vi "UpdateROI.vi"(6 "value":u16, 8 "error in (no error)":errorcluster, 9 "ElementToUpdate":string, 11 "Photometrics Cam v2 in":refnum<class "Photometrics_CH-250_Cam.lvclass">) -> (0 "error out":errorcluster, 3 "Photometrics Cam v2 out":refnum<class "Photometrics_CH-250_Cam.lvclass">)   [LabVIEW 2013, in "Photometrics_CH-250_Cam.lvclass"]
uses:
  Photometrics_CH-250_Cam.lvclass
  CameraSessionClass/CS250-CameraHardwareClass.lvclass
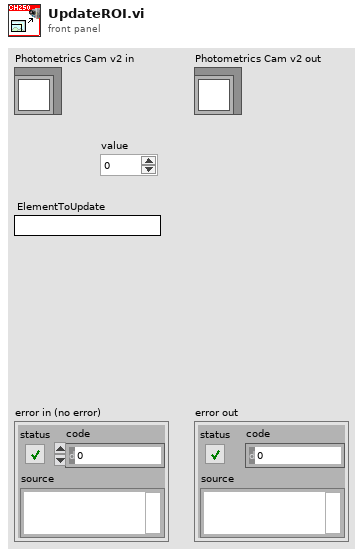
[diagram p1: front panel]
types:
  T1 = typedef "ROI_TypDef.ctl" = cluster{"Width":cluster{"Value":dbl, "Min":dbl, "Max":dbl, "StepSize":dbl, "Tolerance":dbl, "valueactual":dbl}, "Height":cluster{"Value":dbl, "Min":dbl, "Max":dbl, "StepSize":dbl, "Tolerance":dbl, "valueactual":dbl}, "OffsetX":cluster{"Value":dbl, "Min":dbl, "Max":dbl, "StepSize":dbl, "Tolerance":dbl, "valueactual":dbl}, "OffsetY":cluster{"Value":dbl, "Min":dbl, "Max":dbl, "StepSize":dbl, "Tolerance":dbl, "valueactual":dbl}}
  T2 = cluster{"s1":u16, "s2":u16, "sbin":u16, "p1":u16, "p2":u16, "pbin":u16}
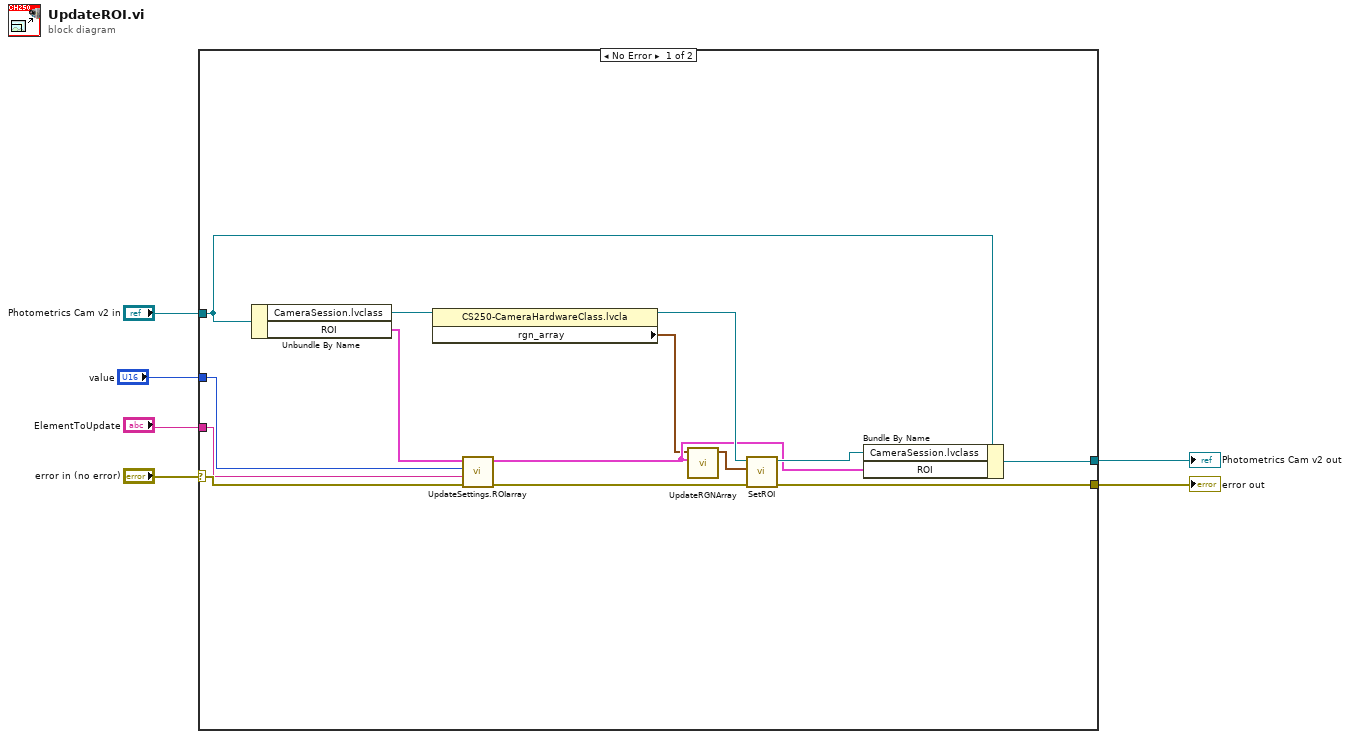
[diagram p0: block diagram]
diagram:
  n1 = case shown="No Error" "error in (no error)" {
    selector: "error in (no error)" -> [w17 w22]
    tunnel: [w20 w21] -> w6
    tunnel: "Photometrics Cam v2 in" -> [w19 w21]
    tunnel: [w18 w22] -> w4
    tunnel: "ElementToUpdate" -> [w11 _]
    tunnel: "value" -> [w10 _]
    frame No Error {
      n2 = Unbundle By Name(w19) -> ("CameraSession.lvclass"=w13:refnum<class "CS250-CameraHardwareClass.lvclass">, "ROI"=w14:T1)
      n3 = property class="CS250-CameraHardwareClass.lvcla"(reference=w13) -> (reference out=w12:refnum<class "CS250-CameraHardwareClass.lvclass">, "rgn_array"=w7:T2)  [unwired: 1 in, 1 out]
      n4 = call "UpdateSettings.ROIarray.vi"("error in (no error)"=w17, "ElementToUpdate"=w11, "value"=w10, "ROI in"=w14) -> ("error out"=w16:errorcluster, "ROI out"=w8:T1)  [unwired: 6 in]
      n5 = call "UpdateRGNArray.vi"("NewROI"=w8, "rgn_array in"=w7) -> ("rgn_array out"=w15:T2)  [unwired: 9 in]
      n6 = call-dynamic "SetROI.vi"("error in (no error)"=w16, "NewROI"=w15, "CameraSession in"=w12) -> ("error out"=w18:errorcluster, "CameraSession out"=w9:refnum<class "CS250-CameraHardwareClass.lvclass">)  [unwired: 7 in]
      n7 = Bundle By Name(cluster=w19, "CameraSession.lvclass"=w9, "ROI"=w8) -> (w20:refnum<class "Photometrics_CH-250_Cam.lvclass">)
    }
    frame Error {
    }
  }
  "Photometrics Cam v2 out" <- w6
  "error out" <- w4
